vi "test_read frame.vi"() -> ()   [LabVIEW 2011]
panel:
  in  "SkipFrame":i32
  out "Image":T1(plugin-control)
  out "FramesPerStim":i32
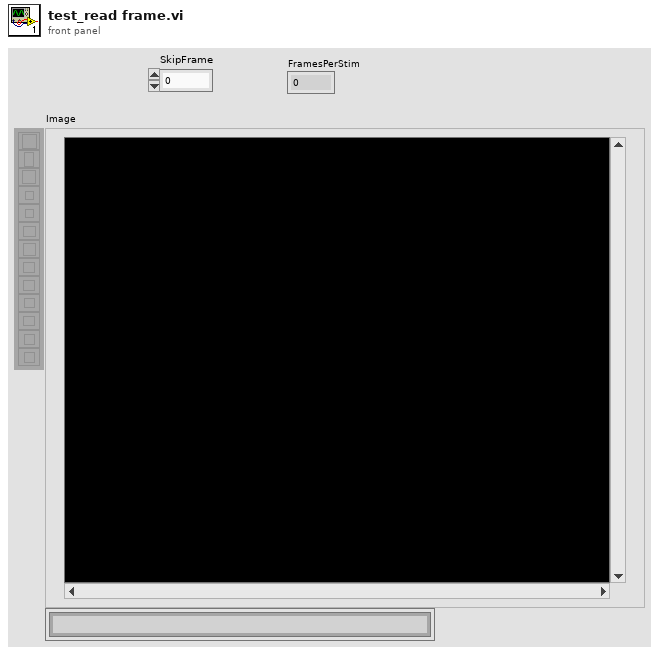
[diagram p1: front panel]
types:
  T1 = typedef "IMAQ Image.ctl" = refnum<image>
  T2 = typedef "Image Type" = u32
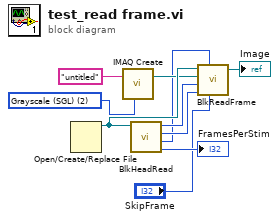
[diagram p0: block diagram]
diagram:
  w7 = T2 2 items=["Grayscale (U8)", "Grayscale (I16)", "Grayscale (SGL)", "Complex (CSG)", "RGB (U32)", "HSL (U32)", "RGB (U64)", "Grayscale (U16)"] ("Image Type")
  n1 = Open/Create/Replace File() -> (refnum out=w9:refnum<file>)  [unwired: 6 in, 2 out]
  n2 = call "IMAQ Create"("Image Name"="untitled", "Image Type"=w7) -> ("New Image"=w6:T1)  [unwired: 3 in, 1 out]
  n3 = call "BlkHeadRead.vi"("引用句柄"=w9) -> ("FramesPerStim"=→"FramesPerStim":i32, "datatype"=w3:i32, "FrameHeight"=w4:i32, "FrameWidth"=w5:i32)  [unwired: 5 in, 2 out]
  n4 = call "BlkReadFrame.vi"("引用句柄输入"=w9, "datatype"=w3, "DST"=w6, "FrameWidth"=w5, "SkipFrame"="SkipFrame", "FrameHeight"=w4) -> ("Image out"=→"Image":T1)  [unwired: 2 in]
